vi "HB_ReadDIO.vi"(8 "error in (no error)":errorcluster, 11 "HBDeviceRef":T1) -> (0 "error out":errorcluster, 2 "All Digital Input Vals":bool[](array[boolean]), 3 "HBDeviceRef":T1)   [LabVIEW 2018]
uses:
  <vilib>/Rock Robotics/WPI/SerialPort/WPI_SerialPortRef.ctl
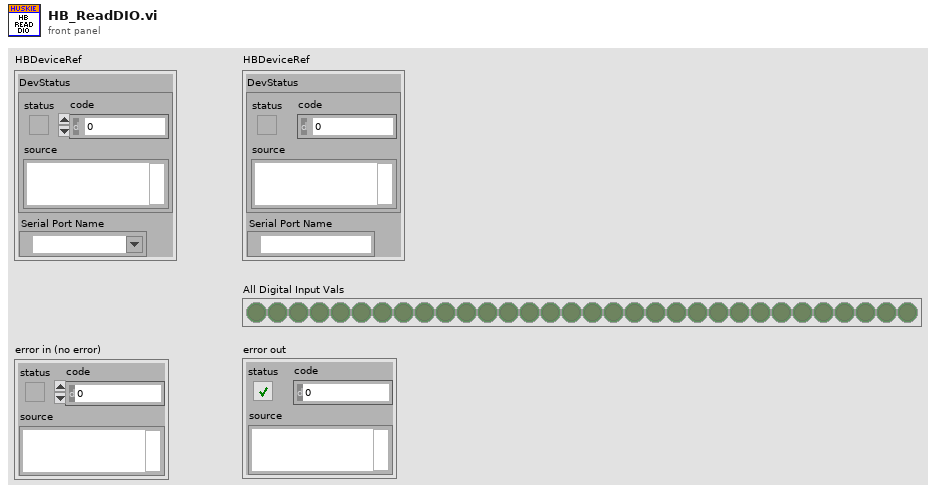
[diagram p1: front panel]
types:
  T1 = typedef "WPI_SerialPortRef.ctl" = cluster{"DevStatus":errorcluster, "Serial Port Name":refnum<visa-resource-name>}
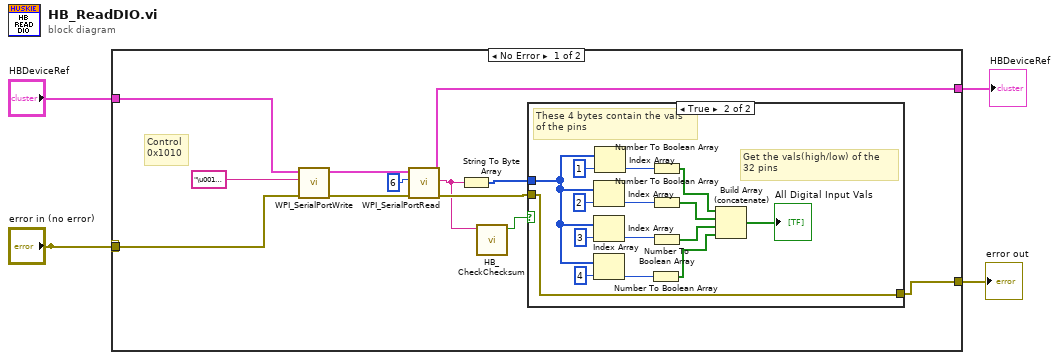
[diagram p0: block diagram]
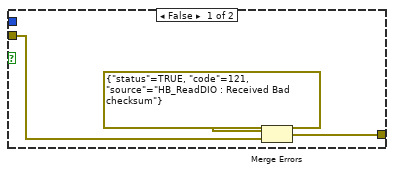
[diagram p2: hidden frame]
diagram:
  n1 = case shown="No Error" "error in (no error)" {
    selector: "error in (no error)" -> [_ w35]
    tunnel: "HBDeviceRef" -> [w16 w36]
    tunnel: [w15 w36] -> w3
    tunnel: "error in (no error)" -> [w14 _]
    tunnel: [w8 w35] -> w2
    frame No Error {
      # "Control\n0x1010"
      n2 = call <vilib>:"WPI_SerialPortWrite.vi"("error in (no error)"=w14, "Buffer"="\u0010\u0010", "SerialPortRef"=w16) -> ("error out"=w12:errorcluster, "SerialPortRef"=w13:T1)  [unwired: 6 in, 1 out]
      n3 = call <vilib>:"WPI_SerialPortRead.vi"("error in (no error)"=w12, "Num Bytes to Read"=u32 6, "SerialPortRef"=w13) -> ("error out"=w9:errorcluster, "Buffer"=w6:string, "SerialPortRef"=w15:T1)  [unwired: 6 in]
      n4 = String To Byte Array(string=w6) -> (unsigned byte array=w7:u8[])
      n5 = call <vilib>:"HB_CheckChecksum.vi"("String"=w6) -> ("Checksum Matches"=w5:bool)  [unwired: 9 in, 1 out]
      n6 = case shown="True" w5 {
        tunnel: w7 -> [_ w21]
        tunnel: w9 -> [w18 w20]
        tunnel: [w17 w20] -> w8
        frame False {
          n7 = Merge Errors(errorcluster {"status"=TRUE, "code"=121, "source"="HB_ReadDIO : Received Bad checksum"} ("error in"), w18) -> (w17:errorcluster)
        }
        frame True {
          # "These 4 bytes contain the vals \nof the pins"
          # "Get the vals(high/low) of the \n32 pins"
          n8 = Index Array(array=w21, index=2) -> (element=w27:u8)
          n9 = Index Array(array=w21, index=3) -> (element=w28:u8)
          n10 = Index Array(array=w21, index=4) -> (element=w29:u8)
          n11 = Index Array(array=w21, index=1) -> (element=w30:u8)
          n12 = Number To Boolean Array(number=w29) -> (Boolean array=w23:bool[])
          n13 = Number To Boolean Array(number=w30) -> (Boolean array=w26:bool[])
          n14 = Number To Boolean Array(number=w27) -> (Boolean array=w25:bool[])
          n15 = Number To Boolean Array(number=w28) -> (Boolean array=w24:bool[])
          n16 = Build Array (concatenate)(w26, w25, w24, w23) -> (→"All Digital Input Vals":bool[])
        }
      }
    }
    frame Error {
    }
  }
  "HBDeviceRef" <- w3
  "error out" <- w2
